vi "macro_WaitAdjust.vi"   [LabVIEW 2019, in "Trajectory_Library.lvlib"]
uses:
  Trajectory_Library.lvlib
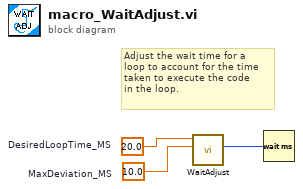
[diagram p0: block diagram]
diagram:
  w2 = 10.0  # MaxDeviation_MS
  w3 = 20.0  # DesiredLoopTime_MS
  # "Adjust the wait time for a\nloop to account for the time\ntaken to execute the code\nin the loop."
  n1 = call "WaitAdjust.vi"("MaxDeviation_MS"=w2, "DesiredLoopTime_MS"=w3) -> ("AdjustedWaitTime_MS"=w1:u32)  [unwired: 8 in, 1 out]
  n2 = Wait (ms)(milliseconds to wait=w1) -> ()  [unwired: 1 out]
